vi "wide milling control.vi"() -> ()   [LabVIEW 2016]
uses:
  <vilib>/SmarAct/MCS/Types/mcsPacket.ctl
  SA driver/test state machine.ctl
  IO/output.ctl
panel:
  in  "number of times to go over table":i32=1
  out "XY Graph":cluster{dbl[], dbl[]}(graph)={[-3000.0, 0.0, 3000.0, 0.0, 3000.0, 0.0, -3000.0, 0.0], [-1500.0, 0.0, -1500.0, 0.0, 1500.0, 0.0, 1500.0, 0.0]}
  out "current digital port states":bool[](array[boolean])
  in  "digital out lines":tag="Dev8/port0/line0:7"
  in  "simulate digital out":bool=TRUE
  out "paused":bool
  in  "ABORT":bool
  out "run finished":bool=TRUE
  out "max steps":i32=4
  in  "resume":bool
  out "current step":i32=4
  in  "reset":bool
  out "stepsize y":dbl=3000.0
  out "final array Y":dbl[](array[numeric])=[-1500.0, -1500.0, 1500.0, 1500.0]
  out "stepsize x":dbl=6000.0
  out "final array X":dbl[](array[numeric])=[-3000.0, 3000.0, 3000.0, -3000.0]
  in  "scan length y [um]":dbl=3000.0 format="%#_13g"
  in  "steps Y":i32=2
  in  "scan length x [um]":dbl=6000.0 format="%#_13g"
  in  "steps X":i32=2
  in  "calc table":bool
  in  "start real":bool
  in  "speed rotation":u32=2000000
  in  "frequency rotation":u32=18000
  in  "speed xy":u32=1000000
  in  "frequency xy":u32=12000
  in  "update speeds":bool
  out "current angle [deg]":dbl format="%.2f"
  out "y position [um]":i32=1500
  out "x position [um]":i32=-3000
  out "y speed":u32=1000000
  out "x speed":u32=1000000
  out "rotation speed":u32=2000000
  out "rotation status":u32
  out "x status":u32
  out "y status":u32
  in  "Home":bool
  in  "revolution":i32
  in  "ROTATE":bool
  in  "MOVE XY":bool
  out "arrived angle":bool
  in  "angle difference deg":i32
  out "current state":enum16{"idle", "running", "fault"}(ring)
  out "arrived xy":bool
  out "packet":T1={"packetType"=enum."SA_POSITION PACKET_TYPE", "channelIndex"=2, "data1"=0, "data2"=1499957, "data3"=0, "data4"=0}
  in  "Position y [um]":i32=1500
  in  "Position x [um]":i32=-3000
  out "Error":errorcluster
  in  "pause":bool
  out "Exit":bool=TRUE
  out "connected":bool=TRUE
  in  "connect":bool
  in  "findSystems":bool caption="Find Systems"
  in  "System locator":string(combo)="usb:id:425839965"
  in  "start sample":bool
  # "A linear positioner with integrated sensor \nshould be connected to channel 0."
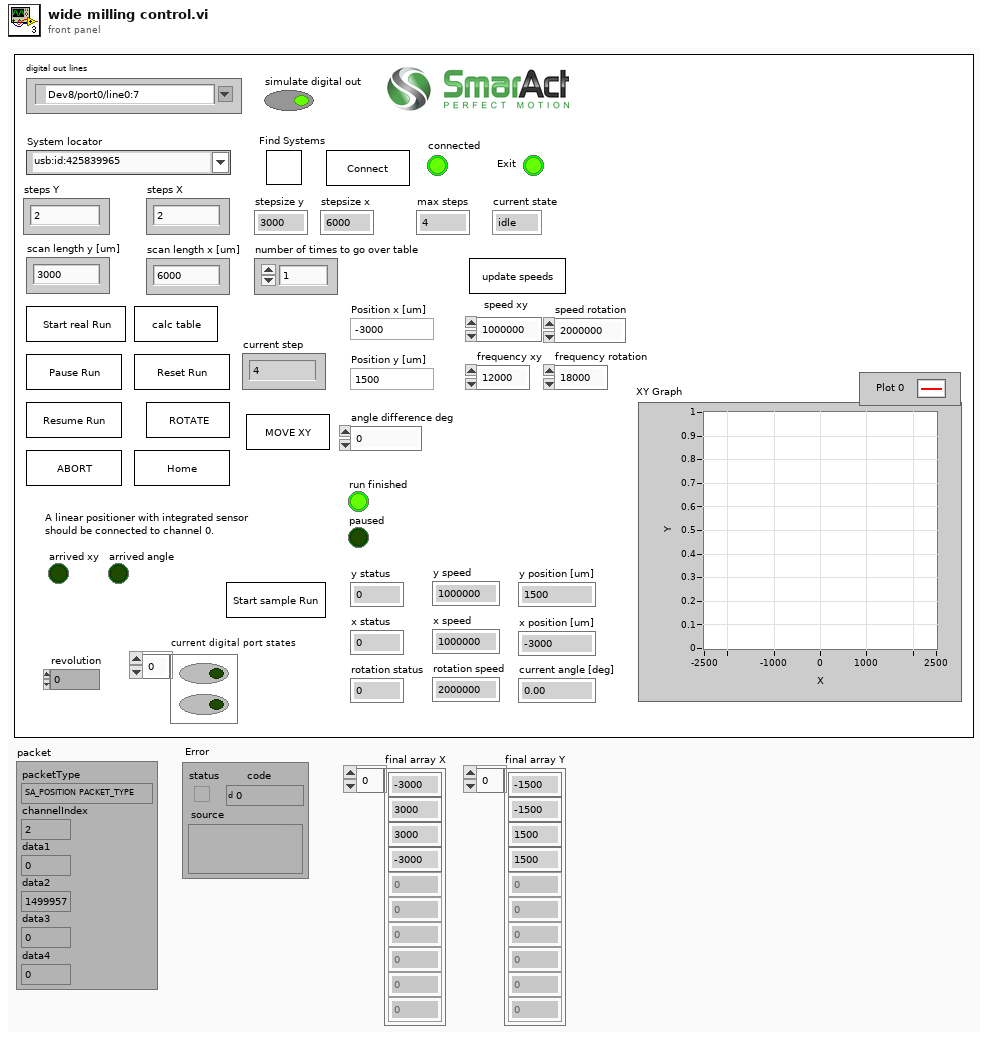
[diagram p1: front panel]
types:
  T1 = typedef "mcsPacket.ctl" = cluster{"packetType":enum32{"SA_NO PACKET_TYPE", "SA_ERROR_ PACKET_TYPE", "SA_POSITION PACKET_TYPE", "SA_COMPLETED PACKET_TYPE", "SA_STATUS PACKET_TYPE", "SA_ANGLE_PACKET_TYPE", "SA_VOLTAGE_LEVEL_PACKET_TYPE", "SA_SENSOR_TYPE_PACKET_TYPE", "SA_SENSOR_ENABLED_PACKET_TYPE", "SA_END_EFFECTOR_TYPE_PACKET_TYPE", "SA_GRIPPER_OPENING_PACKET_TYPE", "SA_FORCE_PACKET_TYPE", "SA_MOVE_SPEED_PACKET_TYPE", "SA_PHYSICAL_POSITION_KNOWN_PACKET_TYPE", "SA_POSITION_LIMIT_PACKET_TYPE", "SA_ANGLE_LIMIT_PACKET_TYPE", "SA_SAFE_DIRECTION_PACKET_TYPE", "SA_SCALE_PACKET_TYPE", "SA_MOVE_ACCELERATION_PACKET_TYPE", "SA_CHANNEL_PROPERTY_PACKET_TYPE", "SA_CAPTURE_BUFFER_PACKET_TYPE", "SA_TRIGGERED_PACKET_TYPE"}, "channelIndex":u32, "data1":u32, "data2":i32, "data3":i32, "data4":u32}
  T2 = typedef "output.ctl" = enum16{"init", "set values", "apply", "read"}
  T3 = typedef "test state machine.ctl" = enum16{"ARRIVED_ROTATE", "ROTATE", "GOTO_XY", "IDLE", "START", "STOP", "ARRIVED_XY", "increment", "check end condition", "GUNS ON", "GUNS OFF"}
  T4 = enum32{"SA_NO PACKET_TYPE", "SA_ERROR_ PACKET_TYPE", "SA_POSITION PACKET_TYPE", "SA_COMPLETED PACKET_TYPE", "SA_STATUS PACKET_TYPE", "SA_ANGLE_PACKET_TYPE", "SA_VOLTAGE_LEVEL_PACKET_TYPE", "SA_SENSOR_TYPE_PACKET_TYPE", "SA_SENSOR_ENABLED_PACKET_TYPE", "SA_END_EFFECTOR_TYPE_PACKET_TYPE", "SA_GRIPPER_OPENING_PACKET_TYPE", "SA_FORCE_PACKET_TYPE", "SA_MOVE_SPEED_PACKET_TYPE", "SA_PHYSICAL_POSITION_KNOWN_PACKET_TYPE", "SA_POSITION_LIMIT_PACKET_TYPE", "SA_ANGLE_LIMIT_PACKET_TYPE", "SA_SAFE_DIRECTION_PACKET_TYPE", "SA_SCALE_PACKET_TYPE", "SA_MOVE_ACCELERATION_PACKET_TYPE", "SA_CHANNEL_PROPERTY_PACKET_TYPE", "SA_CAPTURE_BUFFER_PACKET_TYPE", "SA_TRIGGERED_PACKET_TYPE"}
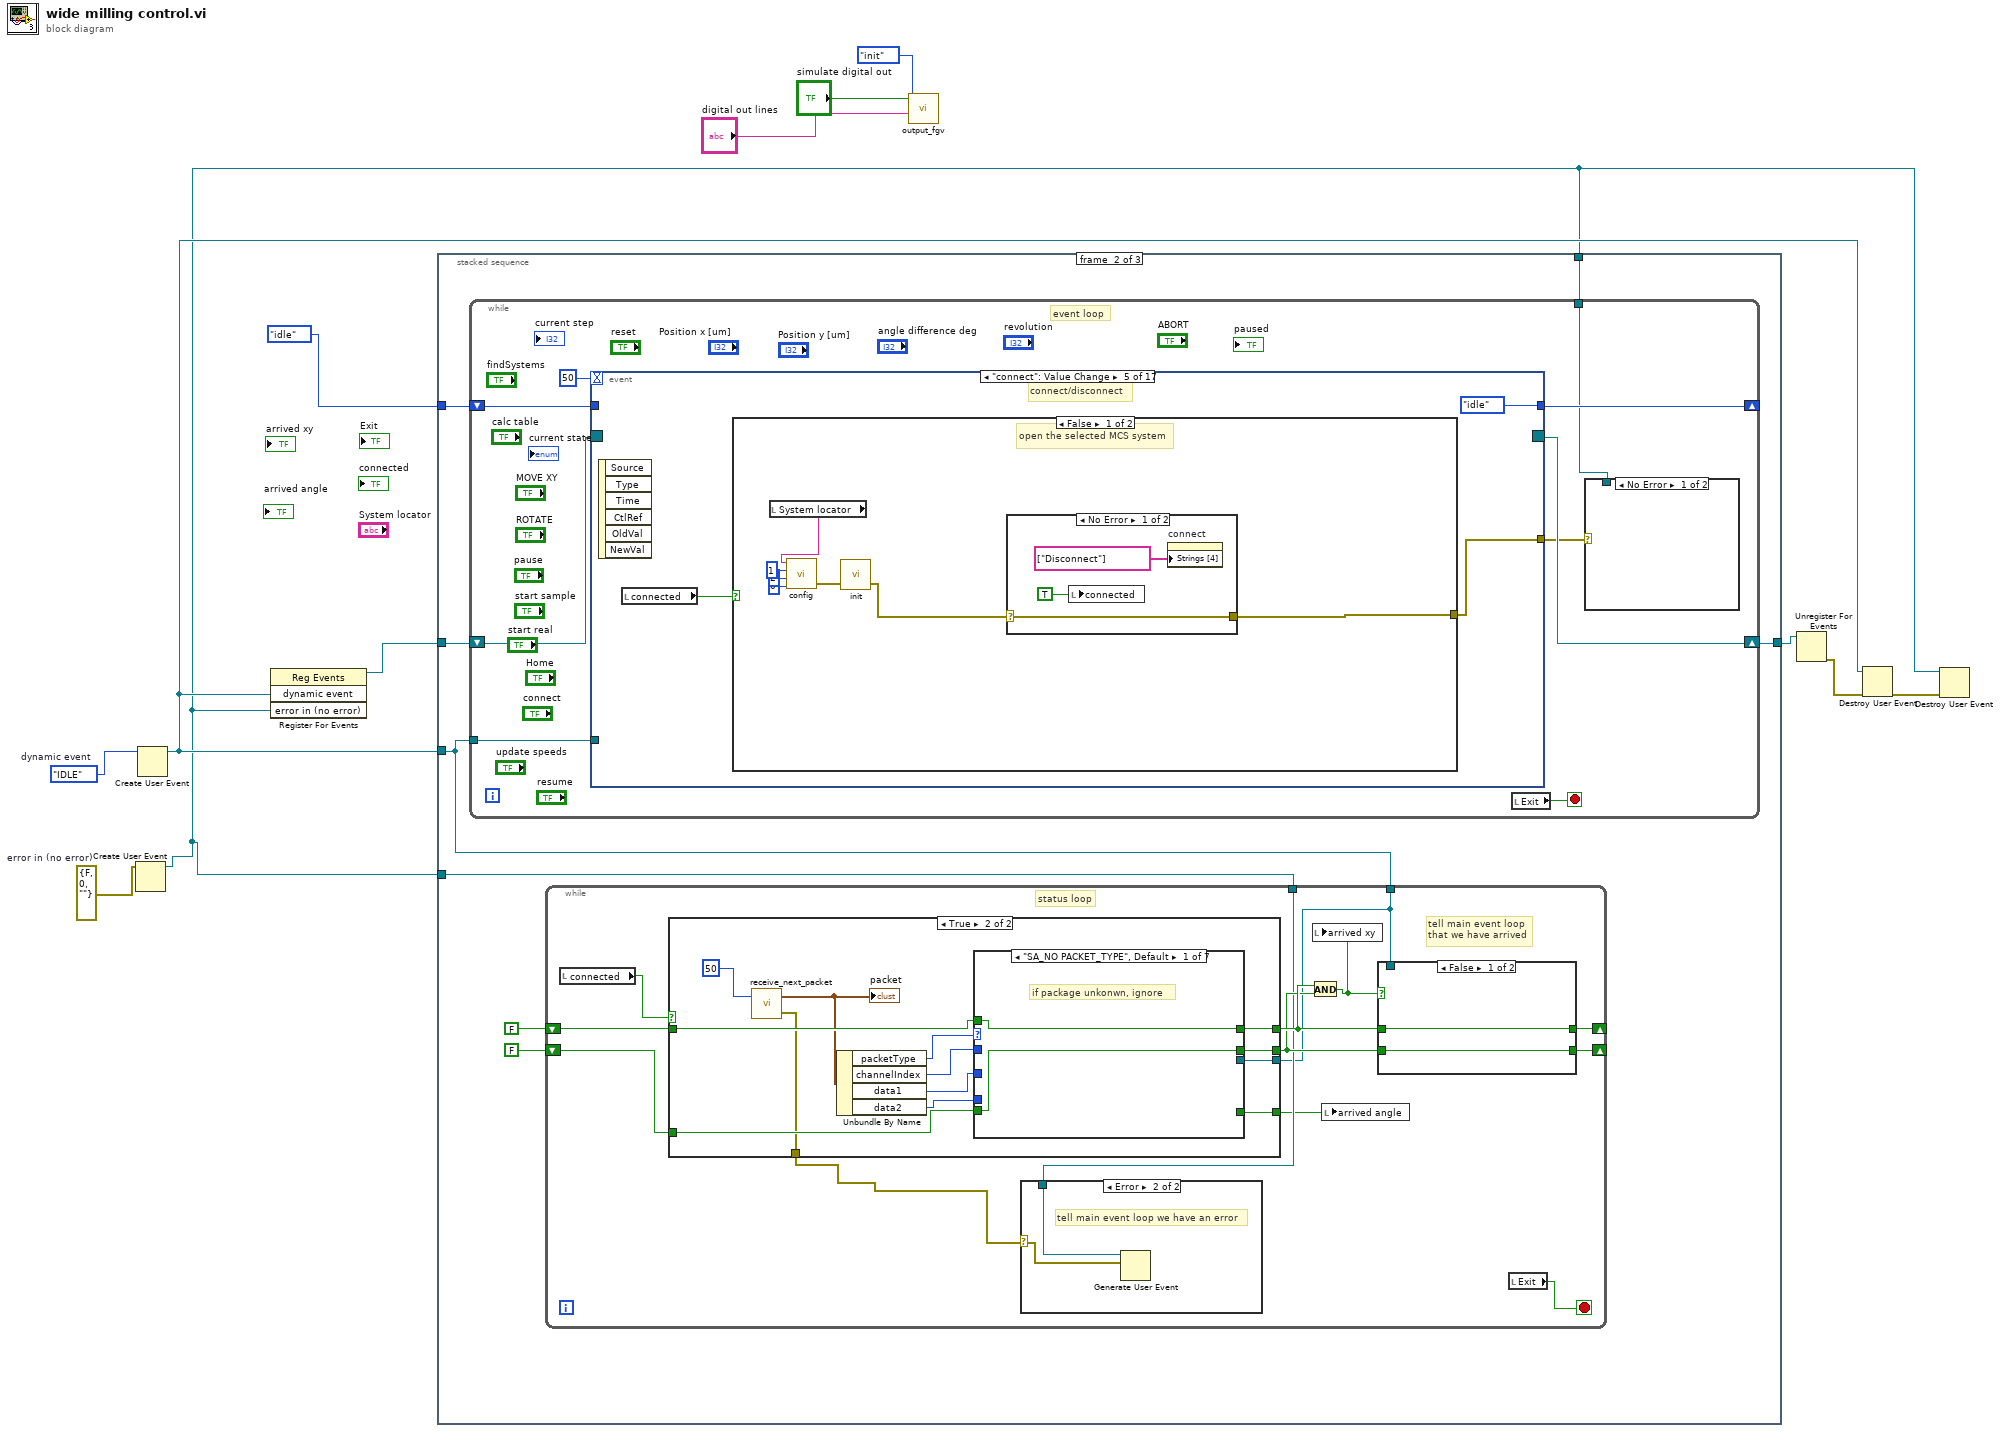
[diagram p0: block diagram]
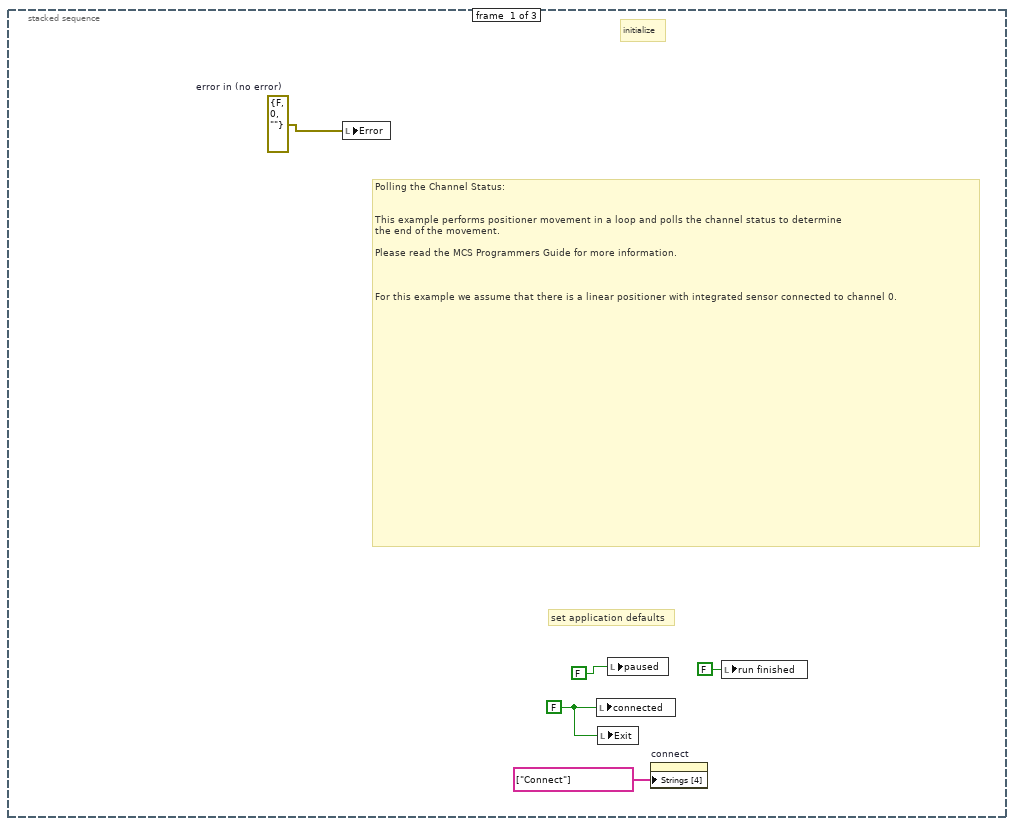
[diagram p2: hidden frame]
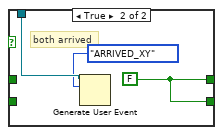
[diagram p4: hidden frame]
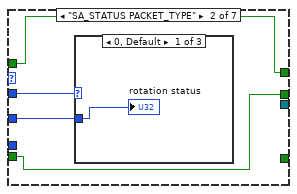
[diagram p6: hidden frame]
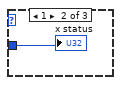
[diagram p7: hidden frame]
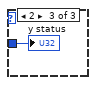
[diagram p8: hidden frame]
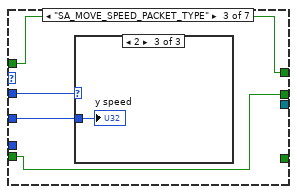
[diagram p9: hidden frame]
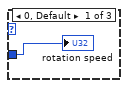
[diagram p10: hidden frame]
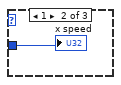
[diagram p11: hidden frame]
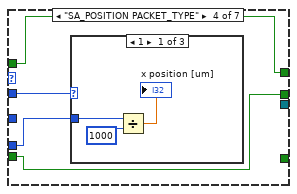
[diagram p12: hidden frame]
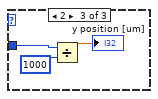
[diagram p14: hidden frame]
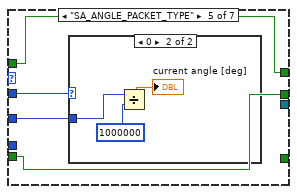
[diagram p15: hidden frame]
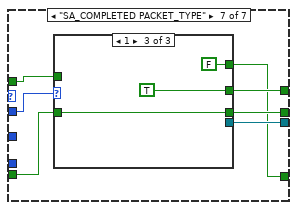
[diagram p18: hidden frame]
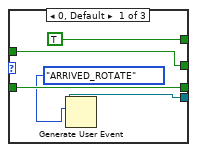
[diagram p19: hidden frame]
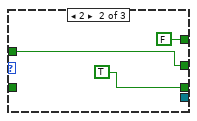
[diagram p20: hidden frame]
diagram:
  w7 = errorcluster {"status"=FALSE, "code"=0, "source"=""}  # error in (no error)
  w9 = test_state_machine."IDLE"  # dynamic event
  n1 = Create User Event(user event datatype=w7) -> (user event=w5:refnum<user-event>)  [unwired: 1 in, 1 out]
  n2 = Create User Event(user event datatype=w9) -> (user event=w8:refnum<user-event>)  [unwired: 1 in, 1 out]
  n3 = register-events(w8, w5) -> (reference out=w12:refnum<event-registration>)  [unwired: 2 in, 1 out]
  n4 = stacked-sequence {
    tunnel: w12 -> [_ w23 _]
    tunnel: [_ w22 _] -> w11
    tunnel: w8 -> [_ w21 _]
    tunnel: w5 -> [_ w20 _]
    tunnel: w5 -> [_ w19 _]
    tunnel: enum16{"idle", "running", "fault"}."idle" ("state") -> [_ w18 _]
    frame #0 {
      w15 = errorcluster {"status"=FALSE, "code"=0, "source"=""}  # error in (no error)
      w17 = FALSE ("connected")
      # "Polling the Channel Status:\n\n\nThis example performs positioner movement in a loop and polls the channel status to determine\nthe end of the movement.\n\nPlease read the MCS Programmers Guide for more information.\n\n\n\nFor this example we assume that there is a linear positioner with integrated sensor connected to channel 0."
      # "set application defaults"
      # "initialize"
      n5 = local write "Error"(w15) -> ()
      n6 = local write "connected"(w17) -> ()
      n7 = local write "Exit"(w17) -> ()
      n8 = local write "paused"(FALSE ("paused 2")) -> ()
      n9 = property on="connect" class="Bool"("Strings [4]"=string[] ["Connect"]) -> ()  [unwired: 2 in, 2 out]
      n10 = local write "run finished"(FALSE ("run finished")) -> ()
    }
    frame #1 {
      n11 = while {
        shift-right: [w119] -> w22
        shift-left: w23 -> [w120]
        tunnel: w21 -> [w118]
        shift-right: [w116] -> _
        shift-left: w18 -> [w117]
        tunnel: w19 -> [w114]
        stop <- w121 stop-if-true
        # "event loop"
        n12 = event shown="[4] \"connect\": Value Change" {
          selector: w120 -> [_ _ _ _ _ _ _ _ _ _ _ _ _ _ _ _ _]
          dyn-events: [_ _ _ _ _ _ _ _ _ _ _ _ _ _ _ _ _] -> w119
          timeout: 50 -> [_ _ _ _ _ _ _ _ _ _ _ _ _ _ _ _ _]
          tunnel: w118 -> [_ w134 w216 w226 _ _ _ w258 _ _ _ _ _ _ _ _ _]
          tunnel: w117 -> [w126 w133 _ _ _ w247 _ _ w262 w268 _ w285 _ w294 w297 w305 w315]
          tunnel: [w126 w132 enum16{"idle", "running", "fault"}."running" ("state") enum16{"idle", "running", "fault"}."running" ("state") enum16{"idle", "running", "fault"}."idle" ("state") w247 _ enum16{"idle", "running", "fault"}."running" ("state") w262 w268 enum16{"idle", "running", "fault"}."idle" ("state") w285 enum16{"idle", "running", "fault"}."idle" ("state") w294 w297 w305 w315] -> w116
          tunnel: [w125 w131 _ w228 w230 _ _ _ _ _ _ w279 _ w293 w298 _ _] -> w115
          event "findSystems": Value Change {
            # "select first locator"
            # "fill the \"System locator\" with\nthe found locators strings"
            # "MCS devices are identified with locator strings.\nThis function writes a list of locator strings of MCS devices that are connected to the PC into \"systemList\". Currently the function only lists MCS with a USB interface."
            # "find systems"
            n13 = event-data() -> ()  [unwired: 1 in, 6 out]
            n14 = call <vilib>:"SA_FindSystems.vi"() -> ("error out"=w130:errorcluster, "systemList"=w129:string[])  [unwired: 10 in]
            n15 = property on="System locator" class="CmbBox"(error in=w130, "Strings[]"=w129) -> (error out=w128:errorcluster)  [unwired: 1 in, 1 out]
            n16 = Index Array(array=w129) -> (element=w127:string)  [unwired: 1 in]
            n17 = property on="System locator" class="CmbBox"(error in=w128, "Value"=w127) -> (error out=w125:errorcluster)  [unwired: 1 in, 1 out]
          }
          event User Event {
            n18 = event-data() -> ("dynamic event"=w135:T3)  [unwired: 1 in, 4 out]
            n19 = case shown="\"running\"" w133 {
              selector: w133 -> [w136 w138]
              tunnel: w135 -> [_ w142]
              tunnel: w134 -> [_ w141]
              tunnel: [w136 w137] -> w132
              tunnel: [_ w139] -> w131
              frame "idle", Default {
                # "idle, remain idle, don't respond to events"
              }
              frame "running" {
                # "running, process events"
                n20 = Wait (ms)(milliseconds to wait=u32 20) -> ()  [unwired: 1 out]
                n21 = case shown="\"GUNS OFF\"" w142 {
                  tunnel: w141 -> [_ _ w151 w162 w174 w178 w187 w190 w203 _]
                  tunnel: [_ w147 w149 w161 w173 w177 w188 w189 _ w211] -> w139
                  tunnel: w138 -> [w143 w146 w148 w152 w164 w176 w186 w192 w202 w210]
                  tunnel: [w143 w146 w148 w152 w164 w176 w186 w192 w201 w210] -> w137
                  frame "IDLE", Default {
                  }
                  frame "GOTO_XY" {
                    n22 = local read "Position y [um]"() -> (w144:i32)
                    n23 = local read "Position x [um]"() -> (w145:i32)
                    n24 = call "Graph As Chart.vi"("Y Value"=w144, "X Value"=w145) -> ()  [unwired: 9 in, 1 out]
                    n25 = call "moveXY.vi"("y position"=w144, "x position"=w145) -> ("error out"=w147:errorcluster)  [unwired: 1 in]
                  }
                  frame "ARRIVED_XY" {
                    n26 = Generate User Event(user event=w151, event data cluster=test_state_machine."GUNS ON" ("event data")) -> (error out=w149:errorcluster)  [unwired: 2 in, 1 out]
                  }
                  frame "GUNS ON" {
                    w153 = TRUE ("single state")
                    # "turn both guns on with signal"
                    n27 = call "output_fgv.vi"("single state"=w153, "index"=0, "action"=output."set values") -> ("error out"=w156:errorcluster)  [unwired: 3 in, 1 out]
                    n28 = call "output_fgv.vi"("single state"=w153, "index"=1, "error in"=w156) -> ("error out"=w155:errorcluster)  [unwired: 3 in, 1 out]
                    n29 = call "output_fgv.vi"("error in"=w155, "action"=output."apply") -> ("error out"=w154:errorcluster)  [unwired: 4 in, 1 out]
                    n30 = Generate User Event(user event=w162, event data cluster=test_state_machine."ROTATE" ("event data"), error in=w154) -> (error out=w161:errorcluster)  [unwired: 1 in, 1 out]
                  }
                  frame "GUNS OFF" {
                    w165 = FALSE ("single state")
                    # "turn both guns off with signal"
                    n31 = call "output_fgv.vi"("single state"=w165, "index"=0, "action"=output."set values") -> ("error out"=w168:errorcluster)  [unwired: 3 in, 1 out]
                    n32 = call "output_fgv.vi"("single state"=w165, "index"=1, "error in"=w168) -> ("error out"=w167:errorcluster)  [unwired: 3 in, 1 out]
                    n33 = call "output_fgv.vi"("error in"=w167, "action"=output."apply") -> ("error out"=w166:errorcluster)  [unwired: 4 in, 1 out]
                    n34 = Generate User Event(user event=w174, event data cluster=test_state_machine."increment" ("event data"), error in=w166) -> (error out=w173:errorcluster)  [unwired: 1 in, 1 out]
                  }
                  frame "ARRIVED_ROTATE" {
                    n35 = Generate User Event(user event=w178, event data cluster=test_state_machine."GUNS OFF" ("event data")) -> (error out=w177:errorcluster)  [unwired: 2 in, 1 out]
                  }
                  frame "START" {
                    n36 = local read "final array X"() -> (w185:dbl[])
                    n37 = local read "final array Y"() -> (w182:dbl[])
                    n38 = local read "current step"() -> (w183:i32)
                    n39 = Index Array(array=w185, index=w183) -> (element=w184:dbl)
                    n40 = Index Array(array=w182, index=w183) -> (element=w181:dbl)
                    n41 = local write "Position x [um]"(w184) -> ()
                    n42 = local write "Position y [um]"(w181) -> ()
                    n43 = Generate User Event(user event=w187, event data cluster=test_state_machine."GOTO_XY" ("event data")) -> (error out=w188:errorcluster)  [unwired: 2 in, 1 out]
                  }
                  frame "increment" {
                    n44 = local read "current step"() -> (w194:i32)
                    n45 = Increment(x=w194) -> (x+1=w193:i32)
                    n46 = local write "current step"(w193) -> ()
                    n47 = Generate User Event(user event=w190, event data cluster=test_state_machine."check end condition" ("event data")) -> (error out=w189:errorcluster)  [unwired: 2 in, 1 out]
                  }
                  frame "check end condition" {
                    # "table finished"
                    # "paused"
                    n48 = local read "current step"() -> (w204:i32)
                    n49 = local read "max steps"() -> (w196:i32)
                    n50 = Decrement(x=w196) -> (x-1=w195:i32)
                    n51 = local read "paused"() -> (w199:bool)
                    n52 = Greater?(x=w204, y=w195) -> (0:w200:bool)
                    "run finished" <- w200
                    n53 = Or(x=w199, y=w200) -> (x .or. y?=w198:bool)
                    n54 = call "Graph As Chart.vi"() -> ("XY Graph"=→"XY Graph":cluster{dbl[], dbl[]})  [unwired: 11 in]
                    n55 = case shown="True" w198 {
                      tunnel: w203 -> [w206 _]
                      tunnel: w202 -> [w205 _]
                      tunnel: [w205 enum16{"idle", "running", "fault"}."idle" ("state")] -> w201
                      frame False {
                        n56 = Generate User Event(user event=w206, event data cluster=test_state_machine."START" ("event data")) -> ()  [unwired: 2 in, 2 out]
                      }
                      frame True {
                        n57 = local write "paused"(FALSE ("paused")) -> ()
                      }
                    }
                  }
                  frame "ROTATE" {
                    n58 = local read "angle difference deg"() -> (w212:i32)
                    n59 = local read "revolution"() -> (w214:i32)
                    n60 = Negate(x=w212) -> (-x=w213:i32)
                    n61 = call "rotate_relative.vi"("angle"=w212, "revolution"=w214) -> ("error out"=w211:errorcluster)  [unwired: 3 in]
                    n62 = local write "angle difference deg"(w213) -> ()
                  }
                }
              }
            }
          }
          event "resume": Value Change {
            n63 = event-data() -> ()  [unwired: 1 in, 6 out]
            n64 = Generate User Event(user event=w216, event data cluster=test_state_machine."START" ("event data")) -> ()  [unwired: 2 in, 2 out]
          }
          event "start real": Value Change {
            n65 = event-data() -> ()  [unwired: 1 in, 6 out]
            n66 = Generate User Event(user event=w226, event data cluster=test_state_machine."START" ("event data")) -> (error out=w228:errorcluster)  [unwired: 2 in, 1 out]
            n67 = local read "final array Y"() -> (w223:dbl[])
            n68 = local read "final array X"() -> (w220:dbl[])
            n69 = local write "current step"(0 ("current step")) -> ()
            n70 = Array Max & Min(array=w223) -> (max value=w222:dbl, min value=w221:dbl)  [unwired: 2 out]
            n71 = Array Max & Min(array=w220) -> (max value=w219:dbl, min value=w218:dbl)  [unwired: 2 out]
            n72 = property on="XY Graph" class="XYGraph (strict)"("XScale.Minimum"=w218) -> ()  [unwired: 2 in, 2 out]
            n73 = property on="XY Graph" class="XYGraph (strict)"("YScale.Minimum"=w221) -> ()  [unwired: 2 in, 2 out]
            n74 = call "Graph As Chart.vi"("Clear Graph?"=TRUE) -> ()  [unwired: 10 in, 1 out]
            n75 = property on="XY Graph" class="XYGraph (strict)"("XScale.Maximum"=w219) -> ()  [unwired: 2 in, 2 out]
            n76 = property on="XY Graph" class="XYGraph (strict)"("YScale.Maximum"=w222) -> ()  [unwired: 2 in, 2 out]
          }
          event "connect": Value Change {
            # "connect/disconnect"
            n77 = event-data() -> ()  [unwired: 1 in, 6 out]
            n78 = local read "connected"() -> (w232:bool)
            n79 = case shown="False" w232 {
              tunnel: [w239 w244] -> w230
              frame False {
                # "open the selected MCS system"
                n80 = local read "System locator"() -> (w237:string)
                n81 = call "config.vi"("System locator"=w237, "X channel"=u32 1, "Y channel"=u32 2, "Rotation channel"=u32 0) -> ("error out"=w238:errorcluster)  [unwired: 1 in]
                n82 = call "init.vi"("error in (no error)"=w238) -> ("error out"=w233:errorcluster)  [unwired: 2 in]
                n83 = case shown="No Error" w233 {
                  selector: w233 -> [w240 w243]
                  tunnel: [w240 w243] -> w239
                  frame No Error {
                    n84 = local write "connected"(TRUE ("connected")) -> ()
                    n85 = property on="connect" class="Bool"("Strings [4]"=string[] ["Disconnect"]) -> ()  [unwired: 2 in, 2 out]
                  }
                  frame Error {
                  }
                }
              }
              frame True {
                # "close the MCS system"
                n86 = call "close.vi"() -> ("error out"=w244:errorcluster)  [unwired: 1 in]
                n87 = local write "connected"(FALSE ("connected")) -> ()
                n88 = property on="connect" class="Bool"("Strings [4]"=string[] ["Connect"]) -> ()  [unwired: 2 in, 2 out]
              }
            }
          }
          event "pause": Value Change {
            # "set pause flag and pause at the end of run"
            # "stop"
            n89 = event-data() -> ()  [unwired: 1 in, 6 out]
            n90 = flat-sequence {
              frame #0 {
                n91 = local write "paused"(TRUE ("paused")) -> ()
              }
            }
          }
          event "ABORT": Value Change {
            w249 = FALSE ("single state")
            n92 = event-data() -> ()  [unwired: 1 in, 6 out]
            n93 = call "output_fgv.vi"("single state"=w249, "index"=0, "action"=output."set values") -> ("error out"=w251:errorcluster)  [unwired: 3 in, 1 out]
            n94 = local read "connected"() -> (w256:bool)
            n95 = call "output_fgv.vi"("single state"=w249, "index"=1, "error in"=w251) -> ("error out"=w250:errorcluster)  [unwired: 3 in, 1 out]
            n96 = case shown="True" w256 {
              frame False {
              }
              frame True {
                n97 = call "stop.vi"() -> ()  [unwired: 1 in, 1 out]
              }
            }
            n98 = call "output_fgv.vi"("error in"=w250, "action"=output."apply") -> ()  [unwired: 4 in, 2 out]
          }
          event "start sample": Value Change {
            # "start move loop"
            n99 = event-data() -> ()  [unwired: 1 in, 6 out]
            n100 = local read "connected"() -> (w259:bool)
            n101 = case shown="True" w259 {
              tunnel: w258 -> [_ w261]
              frame False {
              }
              frame True {
                n102 = Generate User Event(user event=w261, event data cluster=test_state_machine."GOTO_XY" ("event data")) -> ()  [unwired: 2 in, 2 out]
              }
            }
          }
          event "MOVE XY": Value Change {
            # "manually move xy"
            n103 = event-data() -> ()  [unwired: 1 in, 6 out]
            n104 = local read "Position y [um]"() -> (w264:i32)
            n105 = local read "Position x [um]"() -> (w266:i32)
            n106 = call "moveXY.vi"("y position"=w264, "x position"=w266) -> ("error out"=w263:errorcluster)  [unwired: 1 in]
            n107 = Negate(x=w266) -> (-x=w267:i32)
            n108 = Negate(x=w264) -> (-x=w265:i32)
            n109 = local write "Position y [um]"(w265) -> ()
            n110 = local write "Error"(w263) -> ()
            n111 = local write "Position x [um]"(w267) -> ()
          }
          event "ROTATE": Value Change {
            # "manually rotate"
            n112 = event-data() -> ()  [unwired: 1 in, 6 out]
            n113 = local read "angle difference deg"() -> (w269:i32)
            n114 = local read "revolution"() -> (w271:i32)
            n115 = Negate(x=w269) -> (-x=w270:i32)
            n116 = call "rotate_relative.vi"("angle"=w269, "revolution"=w271) -> ()  [unwired: 3 in, 1 out]
            n117 = local write "angle difference deg"(w270) -> ()
          }
          event User Event {
            # "error in polling loop"
            n118 = event-data() -> ("status"=w272:bool, "code"=w273:i32, "source"=w274:string)  [unwired: 1 in, 4 out]
            n119 = Bundle By Name(cluster=errorcluster {"status"=FALSE, "code"=0, "source"=""} ("Error"), "status"=w272, "code"=w273, "source"=w274) -> (w276:errorcluster)
            n120 = local write "Exit"(w272) -> ()
            n121 = call <vilib>:"Simple Error Handler.vi"("error in (no error)"=w276) -> ("error out"=→"Error":errorcluster)  [unwired: 4 in, 4 out]
          }
          event "Home": Value Change {
            # "home xy and rotation to a known starting point"
            n122 = event-data() -> ()  [unwired: 1 in, 6 out]
            n123 = local read "revolution"() -> (w283:i32)
            n124 = call "moveXY.vi"("y position"=0, "x position"=0) -> ("error out"=w282:errorcluster)  [unwired: 1 in]
            n125 = call "rotate_absolute.vi"("error in (no error)"=w282, "angle"=w283, "revolution"=0) -> ("error out"=w279:errorcluster)  [unwired: 2 in]
          }
          event Panel Close? {
            # "NOTE:\nMake sure not to use the red \"Abort Execution\" button in the\nLabVIEW menu to abort the application execution.\nDoing so will not close the device connection with the consequence that\na re-open after the next application start will fail."
            # "\"Panel Close\" (\"X\") was clicked by the user:\nWe discard the close command and set an \"exit\" flag. This gives us the change to proper disconnect the device and clean up the application before closing the window."
            # "window \"X\" (close)"
            n126 = event-data() -> ()  [unwired: 1 in, 4 out]
            n127 = local write "Exit"(TRUE ("exit")) -> ()
            n128 = event-data("Discard?"=TRUE) -> ()  [unwired: 1 in, 1 out]
          }
          event Timeout {
            # "non time critical items go here"
            # "update these values from received packages"
            n129 = event-data() -> ()  [unwired: 1 in, 3 out]
            n130 = call "output_fgv.vi"("action"=output."read") -> ("current valve states"=→"current digital port states":bool[])  [unwired: 5 in, 1 out]
            n131 = local read "connected"() -> (w292:bool)
            n132 = case shown="False" w292 {
              tunnel: [_ w296] -> w293
              frame False {
              }
              frame True {
                n133 = call "get_speeds_and_positions.vi"() -> ("error out"=w295:errorcluster)  [unwired: 1 in]
                n134 = call "get_status.vi"("error in (no error)"=w295) -> ("error out"=w296:errorcluster)
              }
            }
            n135 = call "output_fgv.vi"("action"=output."apply") -> ()  [unwired: 5 in, 2 out]
          }
          event "update speeds": Value Change {
            n136 = event-data() -> ()  [unwired: 1 in, 6 out]
            n137 = call "set_speeds.vi"("speed rotation"="speed rotation", "frequency rotation"="frequency rotation", "speed xy"="speed xy", "frequency xy"="frequency xy") -> ("error out"=w298:errorcluster)  [unwired: 1 in]
          }
          event "calc table": Value Change {
            n138 = event-data() -> ()  [unwired: 1 in, 6 out]
            n139 = call "calculateTableSimpleSerpentine.vi"("scan length y"="scan length y [um]", "number of times to go over table"="number of times to go over table", "steps Y"="steps Y", "scan length x"="scan length x [um]", "steps X"="steps X") -> ("stepsize y"=→"stepsize y":dbl, "final array Y"=→"final array Y":dbl[], "stepsize x"=→"stepsize x":dbl, "final array X"=→"final array X":dbl[], "size x"=→"max steps":i32)
          }
          event "reset": Value Change {
            n140 = event-data() -> ()  [unwired: 1 in, 6 out]
            n141 = local write "current step"(0 ("current step")) -> ()
          }
        }
        n142 = local read "Exit"() -> (w121:bool)
        n143 = case shown="No Error" w115 {
          selector: w115 -> [_ w124]
          tunnel: w114 -> [_ w123]
          frame No Error {
          }
          frame Error {
            n144 = Generate User Event(user event=w123, event data cluster=w124) -> ()  [unwired: 2 in, 2 out]
          }
        }
      }
      n145 = while {
        shift-right: [w35] -> _
        shift-left: FALSE -> [w37]
        shift-right: [w33] -> _
        shift-left: FALSE -> [w36]
        tunnel: w21 -> [w30]
        tunnel: w20 -> [w31]
        stop <- w38 stop-if-true
        # "tell main event loop\nthat we have arrived"
        # "status loop"
        n146 = local read "connected"() -> (w27:bool)
        n147 = case shown="True" w27 {
          tunnel: [w47 w57] -> w34
          tunnel: w37 -> [w47 w56]
          tunnel: [w46 w55] -> w32
          tunnel: w36 -> [w46 w54]
          tunnel: [_ w53] -> w26
          tunnel: w30 -> [_ w52]
          tunnel: [_ w51] -> w28
          frame False {
            # "no error"
          }
          frame True {
            n148 = call "receive_next_packet.vi"("timeout"=u32 50) -> ("error out"=w53:errorcluster, "packet"=w49:T1)  [unwired: 1 in]
            "packet" <- w49
            n149 = Unbundle By Name(w49) -> ("packetType"=w59:T4, "channelIndex"=w58:u32, "data1"=w50:u32, "data2"=w48:i32)
            n150 = case shown="\"SA_NO PACKET_TYPE\", Default" w59 {
              tunnel: w58 -> [_ w66 w73 w80 w90 _ w101]
              tunnel: [w62 w64 w71 w79 w88 w95 w102] -> w57
              tunnel: w56 -> [w62 w64 w71 w79 w88 w95 w100]
              tunnel: [w61 w63 w70 w78 w87 w94 w99] -> w55
              tunnel: w54 -> [w61 w63 w70 w78 w87 w94 w98]
              tunnel: w52 -> [_ _ _ _ _ _ w97]
              tunnel: [_ _ _ _ _ _ w96] -> w51
              tunnel: w50 -> [_ w65 w72 _ w89 _ _]
              tunnel: w48 -> [_ _ _ w77 _ _ _]
              frame "SA_NO PACKET_TYPE", Default {
                # "if package unkonwn, ignore"
              }
              frame "SA_STATUS PACKET_TYPE" {
                n151 = case shown="0, Default" w66 {
                  tunnel: w65 -> [w67 w68 w69]
                  frame 0, Default {
                    "rotation status" <- w67
                  }
                  frame 1 {
                    "x status" <- w68
                  }
                  frame 2 {
                    "y status" <- w69
                  }
                }
              }
              frame "SA_MOVE_SPEED_PACKET_TYPE" {
                n152 = case shown="2" w73 {
                  tunnel: w72 -> [w74 w75 w76]
                  frame 0, Default {
                    "rotation speed" <- w74
                  }
                  frame 1 {
                    "x speed" <- w75
                  }
                  frame 2 {
                    "y speed" <- w76
                  }
                }
              }
              frame "SA_POSITION PACKET_TYPE" {
                n153 = case shown="1" w80 {
                  tunnel: w77 -> [w83 _ w85]
                  frame 1 {
                    n154 = Divide(x=w83, y=1000) -> (x/y=→"x position [um]":dbl)
                  }
                  frame 0, Default {
                  }
                  frame 2 {
                    n155 = Divide(x=w85, y=1000) -> (x/y=→"y position [um]":dbl)
                  }
                }
              }
              frame "SA_ANGLE_PACKET_TYPE" {
                n156 = case shown="0" w90 {
                  tunnel: w89 -> [_ w93]
                  frame 1, Default {
                  }
                  frame 0 {
                    n157 = Divide(x=w93, y=u32 1000000) -> (x/y=→"current angle [deg]":dbl)
                  }
                }
              }
              frame "SA_ERROR_ PACKET_TYPE" {
              }
              frame "SA_COMPLETED PACKET_TYPE" {
                n158 = case shown="1" w101 {
                  tunnel: [w106 w109 TRUE] -> w102
                  tunnel: w100 -> [w106 w109 _]
                  tunnel: [w107 TRUE w112] -> w99
                  tunnel: w98 -> [w107 _ w112]
                  tunnel: w97 -> [w105 _ _]
                  tunnel: [TRUE ("arrived angle") FALSE ("arrived angle") FALSE ("arrived angle")] -> w96
                  frame 0, Default {
                    n159 = Generate User Event(user event=w105, event data cluster=test_state_machine."ARRIVED_ROTATE" ("event data")) -> ()  [unwired: 2 in, 2 out]
                  }
                  frame 2 {
                  }
                  frame 1 {
                  }
                }
              }
            }
          }
        }
        n160 = case shown="Error" w26 {
          selector: w26 -> [_ w40]
          tunnel: w31 -> [_ w39]
          frame No Error {
          }
          frame Error {
            # "tell main event loop we have an error"
            n161 = Generate User Event(user event=w39, event data cluster=w40) -> ()  [unwired: 2 in, 2 out]
          }
        }
        n162 = And(x=w34, y=w32) -> (x .and. y?=w29:bool)
        n163 = local write "arrived xy"(w29) -> ()
        n164 = local write "arrived angle"(w28) -> ()
        n165 = case shown="False" w29 {
          tunnel: [w42 w45] -> w35
          tunnel: w34 -> [w42 _]
          tunnel: [w41 w45] -> w33
          tunnel: w32 -> [w41 _]
          tunnel: w30 -> [_ w44]
          frame False {
          }
          frame True {
            w45 = FALSE
            # "both arrived"
            n166 = Generate User Event(user event=w44, event data cluster=test_state_machine."ARRIVED_XY" ("event data")) -> ()  [unwired: 2 in, 2 out]
          }
        }
        n167 = local read "Exit"() -> (w38:bool)
      }
    }
    frame #2 {
      # "clean up"
      n168 = local read "connected"() -> (w316:bool)
      n169 = case shown="True" w316 {
        frame False {
        }
        frame True {
          # "always make sure to close the connection\nto the device before quitting the program"
          n170 = call "close.vi"() -> ("error out"=w317:errorcluster)  [unwired: 1 in]
          n171 = call <vilib>:"Clear Errors.vi"("error in (no error)"=w317) -> ()  [unwired: 5 in, 2 out]
        }
      }
    }
  }
  n172 = call "output_fgv.vi"("Line(s)"="digital out lines", "action"=output."init", "simulate"="simulate digital out") -> ()  [unwired: 3 in, 2 out]
  n173 = Unregister For Events(event registration refnum=w11) -> (error out=w10:errorcluster)  [unwired: 1 in]
  n174 = Destroy User Event(user event=w8, error in=w10) -> (error out=w6:errorcluster)
  n175 = Destroy User Event(user event=w5, error in=w6) -> ()  [unwired: 1 out]
